vi "NXT_ Init Motor Data.vi"() -> (0 "_motorData":T1)   [LabVIEW 2012, in "Tugboat.lvrbt"]
uses:
  Tugboat.lvrbt
  motorData_t.ctl
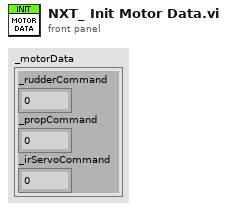
[diagram p1: front panel]
types:
  T1 = typedef "motorData_t.ctl" = cluster{"_rudderCommand":u16, "_propCommand":u16, "_irServoCommand":u16}
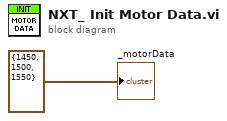
[diagram p0: block diagram]
diagram:
  "_motorData" <- T1 {"_rudderCommand"=1450, "_propCommand"=1500, "_irServoCommand"=1550} ("_motorData")
